vi "Audio.Trim Waveform.vi"(5 "Len":i32=44100, 7 "Max Delay":dbl=0.06 format="%#_13g", 10 "Threshold":dbl=0.01, 11 "Data In":waveform(dbl)(graph)={"t0"=timestamp(3623763314.3865924 s since 1904-01-01), "dt"=2.2675736961451248e-05, "Y"=array[48508 elements]}) -> (3 "Data Out":waveform(dbl)(graph))   [LabVIEW 2018]
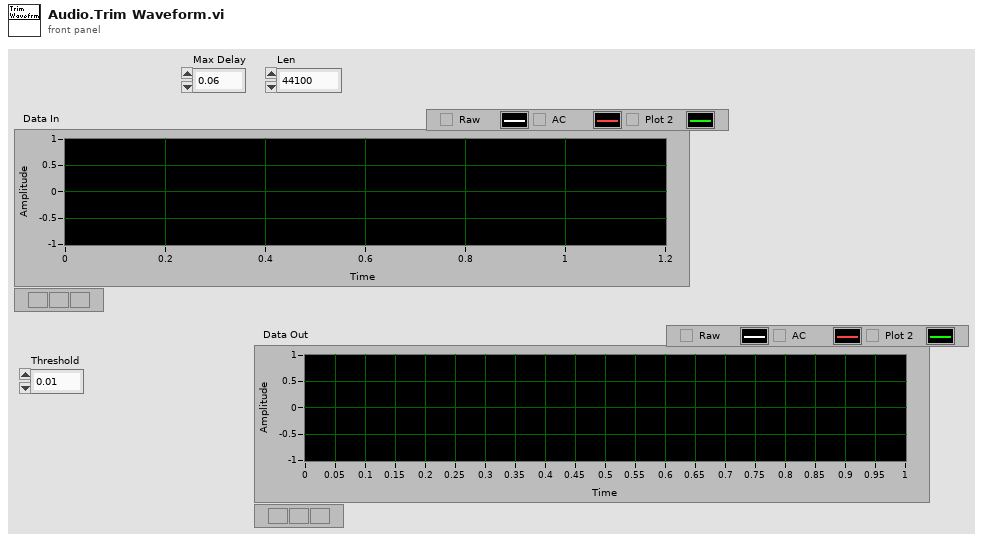
[diagram p1: front panel]
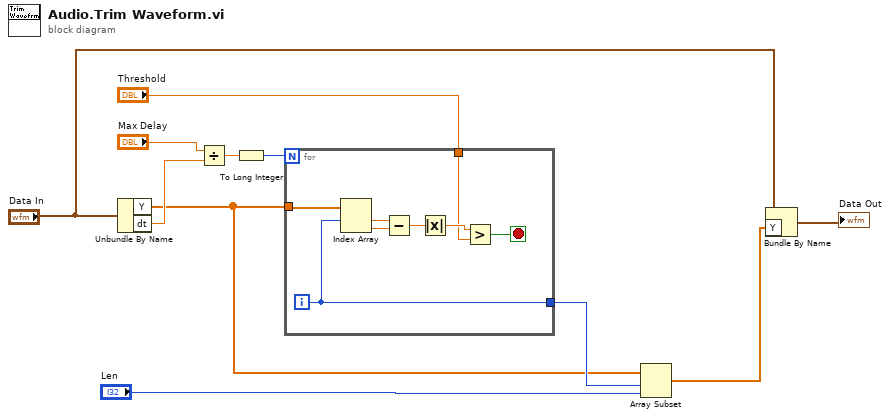
[diagram p0: block diagram]
diagram:
  n1 = Unbundle By Name("Data In") -> ("Y"=w4:dbl[], "dt"=w10:dbl)
  n2 = Divide(x="Max Delay", y=w10) -> (x/y=w9:dbl)
  n3 = To Long Integer(number=w9) -> (32bit integer=w8:i32)
  n4 = for {
    N: w8 -> [_]
    tunnel: w4 -> [w19]
    tunnel: "Threshold" -> [w13]
    tunnel: [w12] -> w6
    i -> [w12]
    stop <- w14 stop-if-true
    n5 = Index Array(array=w19, index #1=w12) -> (element #1=w17:dbl, element #2=w18:dbl)  [unwired: 1 in]
    n6 = Subtract(x=w17, y=w18) -> (x-y=w16:dbl)
    n7 = Absolute Value(x=w16) -> (abs(x)=w15:dbl)
    n8 = Greater?(x=w15, y=w13) -> (0:w14:bool)
  }
  n9 = Array Subset(array=w4, index=w6, length="Len") -> (w2:dbl[])
  n10 = Bundle By Name(cluster="Data In", "Y"=w2) -> (→"Data Out":waveform(dbl))
